vi "Auto Scorer.vi"() -> ()   [LabVIEW 2024, in "Word Search Scorer.lvlib"]
uses:
  Word Search Scorer.lvlib
  Scorer State.ctl
  Scoring Result.ctl
panel:
  out "Response":string
  out "Scoring Result":T1
  out "Run Time":dbl format="%<%M:%S%1u>t"
  out "Run Start":timestamp
  out "VI Refnum":refnum<vi>
  out "App Ref":refnum<vi>
  out "Zip":path
  out "Upload Error":errorcluster
  out "Score Error":errorcluster
  out "Download Error":errorcluster
  out "Poll Error":errorcluster
  out "Last Poll":timestamp format="%<%Y-%m-%d %H:%M:%S>T"
  out "State":T2
  out "Previous Submission":i32
  out "Current Submission":i32
  out "Time to next poll":dbl format="%#.0f"
  in  "Poll Period":dbl=60.0
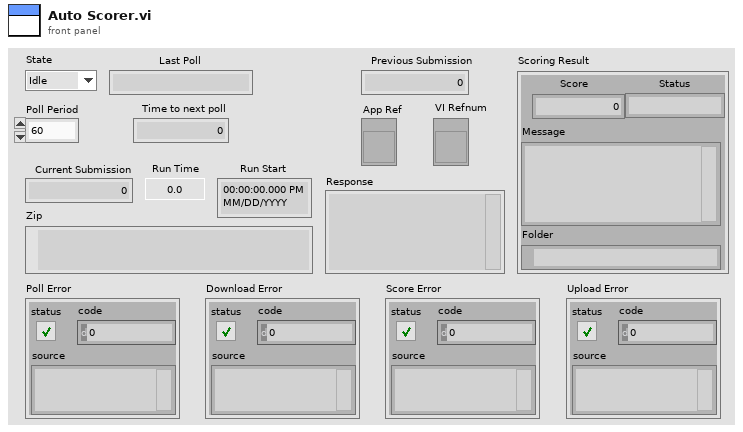
[diagram p1: front panel]
types:
  T1 = typedef "Word Search Scorer.lvlib/Scoring Result.ctl" = cluster{"Score":dbl, "Status":string, "Message":string, "Folder":path}
  T2 = typedef "Word Search Scorer.lvlib/Scorer State.ctl" = enum16{"Idle", "Poll", "Run", "Upload", "Error", "Timeout"}
  T3 = enum32{"Bad", "Idle", "Run top level", "Running"}
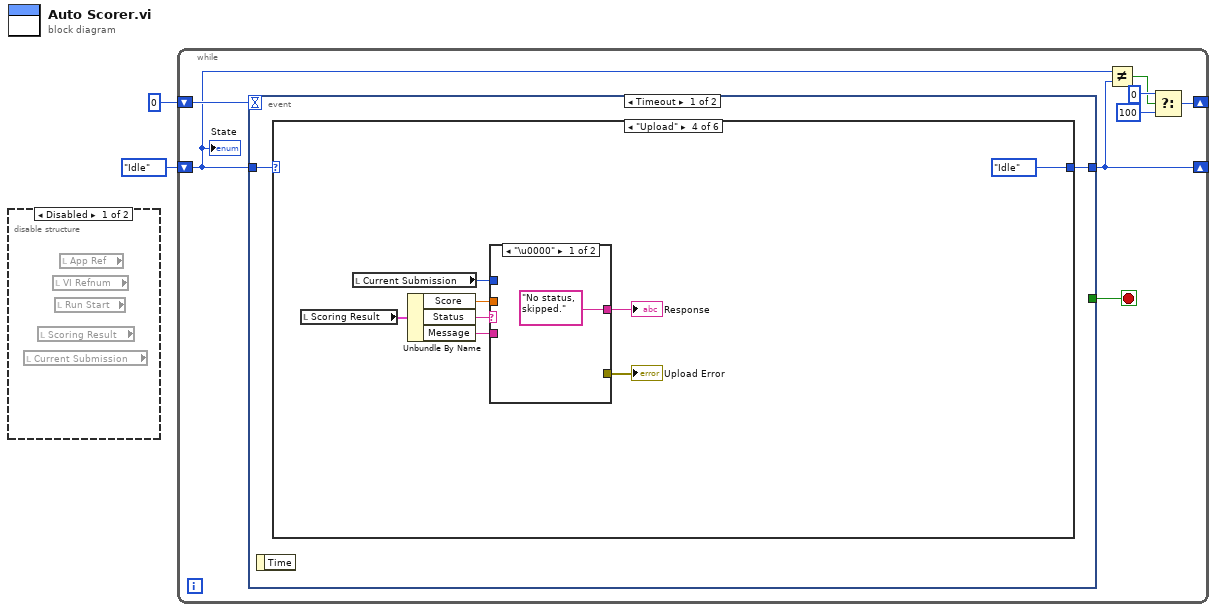
[diagram p0: block diagram]
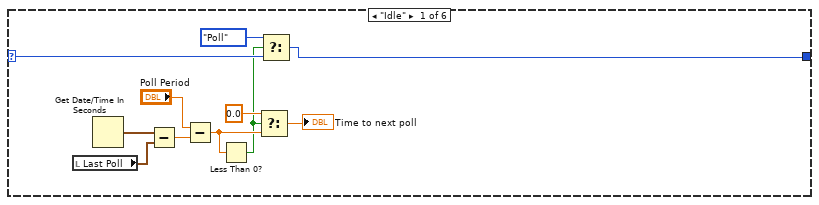
[diagram p3: hidden frame]
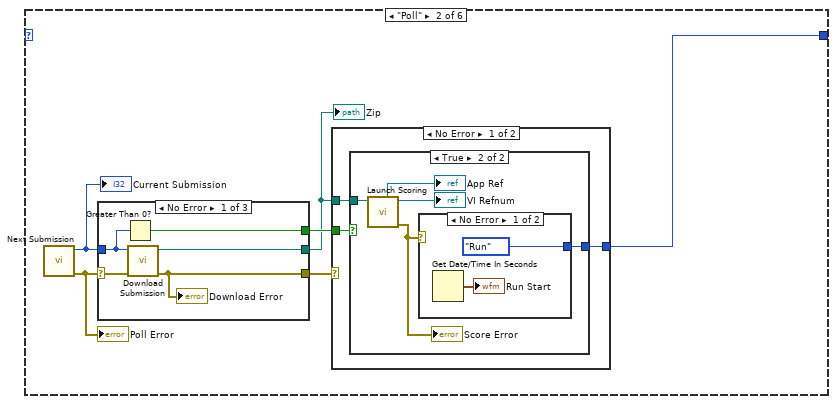
[diagram p4: hidden frame]
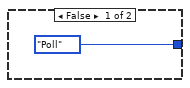
[diagram p5: hidden frame]
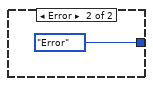
[diagram p6: hidden frame]
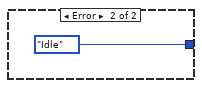
[diagram p7: hidden frame]
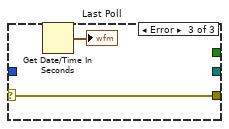
[diagram p9: hidden frame]
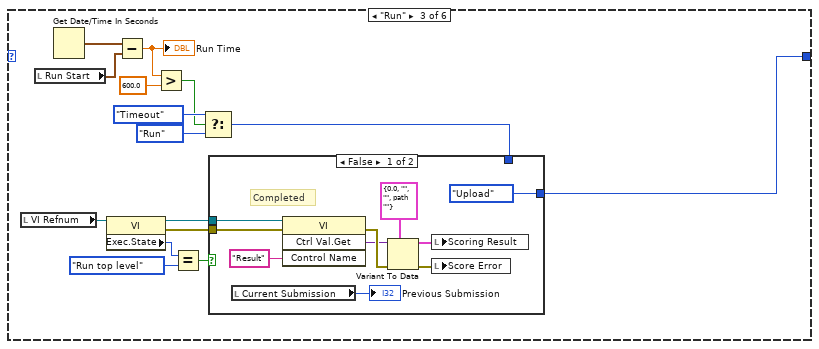
[diagram p10: hidden frame]
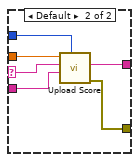
[diagram p12: hidden frame]
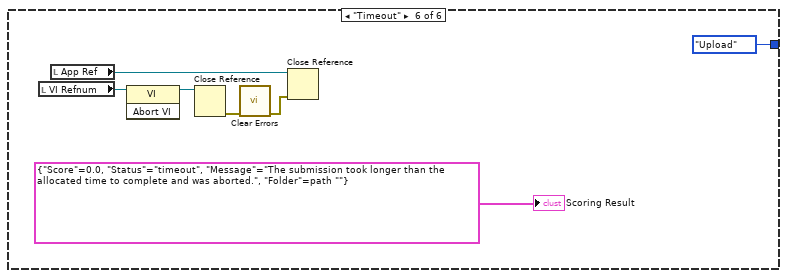
[diagram p14: hidden frame]
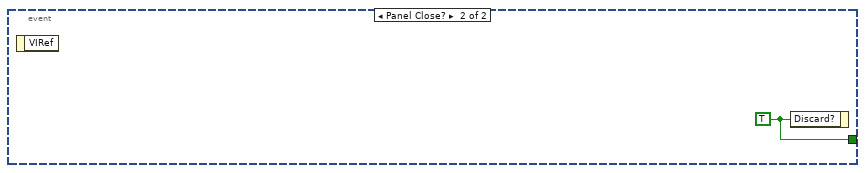
[diagram p15: hidden frame]
diagram:
  n1 = disable-structure shown="Disabled" {
    frame Disabled {
      n2 = local read "Current Submission"() -> ()  [unwired: 1 out]
      n3 = local read "Scoring Result"() -> ()  [unwired: 1 out]
      n4 = local read "VI Refnum"() -> ()  [unwired: 1 out]
      n5 = local read "Run Start"() -> ()  [unwired: 1 out]
      n6 = local read "App Ref"() -> ()  [unwired: 1 out]
    }
    frame Enabled {
    }
  }
  n7 = while {
    shift-right: [w9] -> _
    shift-left: Scorer_State."Idle" ("Scorer State") -> [w8]
    shift-right: [w6] -> _
    shift-left: 0 -> [w10]
    stop <- w3 stop-if-true
    n8 = event shown="[0] Timeout" {
      selector: _ -> [_ _]
      dyn-events: _ -> [_ _]
      timeout: w10 -> [_ _]
      tunnel: w8 -> [w12 _]
      tunnel: [w11 _] -> w9
      tunnel: [_ w100] -> w3
      event Timeout {
        n9 = event-data() -> ()  [unwired: 1 in, 1 out]
        n10 = case shown="\"Upload\"" w12 {
          selector: w12 -> [w16 _ _ _ w92 _]
          tunnel: [w13 w26 w59 Scorer_State."Idle" ("Scorer State") w92 Scorer_State."Upload" ("Scorer State")] -> w11
          frame "Idle" {
            n11 = local read "Last Poll"() -> (w22:timestamp)
            n12 = Get Date/Time In Seconds() -> (seconds since 1Jan1904=w23:timestamp)
            n13 = Subtract(x=w23, y=w22) -> (x-y=w21:dbl)
            n14 = Subtract(x="Poll Period", y=w21) -> (x-y=w19:dbl)
            n15 = Less Than 0?(x=w19) -> (x < 0?=w15:bool)
            n16 = Select(t=0.0, s=w15, f=w19) -> (s? t:f=→"Time to next poll":dbl)
            n17 = Select(t=Scorer_State."Poll", s=w15, f=w16) -> (s? t:f=w13:T2)
          }
          frame "Poll" {
            n18 = call "Next Submission.vi"() -> ("error out"=w28:errorcluster, "submission"=w24:i32)  [unwired: 9 in, 1 out]
            "Poll Error" <- w28
            "Current Submission" <- w24
            n19 = case shown="No Error" w28 {
              selector: w28 -> [w46 w48 w49]
              tunnel: w24 -> [w47 _ _]
              tunnel: [w45 _ _] -> w25
              tunnel: [w44 w48 w49] -> w29
              tunnel: [w43 _ _] -> w27
              frame No Error {
                n20 = Greater Than 0?(x=w47) -> (x > 0?=w43:bool)
                n21 = call "Download Submission.vi"("error in (no error)"=w46, "submission"=w47) -> ("error out"=w44:errorcluster, "Zip Path"=w45:path)  [unwired: 7 in, 1 out]
                "Download Error" <- w44
              }
              frame Default {
              }
              frame Error {
                # "No submissions"
                n22 = Get Date/Time In Seconds() -> (seconds since 1Jan1904=→"Last Poll":timestamp)
              }
            }
            "Zip" <- w25
            n23 = case shown="No Error" w29 {
              tunnel: w27 -> [w32 _]
              tunnel: [w31 Scorer_State."Idle" ("Scorer State")] -> w26
              tunnel: w25 -> [w30 _]
              frame No Error {
                n24 = case shown="True" w32 {
                  tunnel: [Scorer_State."Poll" ("Scorer State") w37] -> w31
                  tunnel: w30 -> [_ w34]
                  frame False {
                  }
                  frame True {
                    n25 = call "Launch Scoring.vi"("Zip"=w34) -> ("error out"=w38:errorcluster, "VI Refnum"=→"VI Refnum":refnum<vi>, "App Ref"=→"App Ref":refnum<vi>)  [unwired: 8 in]
                    "Score Error" <- w38
                    n26 = case shown="No Error" w38 {
                      tunnel: [Scorer_State."Run" ("Scorer State") Scorer_State."Error" ("Scorer State")] -> w37
                      frame No Error {
                        n27 = Get Date/Time In Seconds() -> (seconds since 1Jan1904=→"Run Start":timestamp)
                      }
                      frame Error {
                      }
                    }
                  }
                }
              }
              frame Error {
              }
            }
          }
          frame "Run" {
            n28 = local read "VI Refnum"() -> (w65:refnum<vi>)
            n29 = local read "Run Start"() -> (w61:timestamp)
            n30 = Get Date/Time In Seconds() -> (seconds since 1Jan1904=w62:timestamp)
            n31 = property class="VI"(reference=w65) -> (reference out=w52:refnum<vi>, error out=w51:errorcluster, "Exec.State"=w64:T3)  [unwired: 1 in]
            n32 = Subtract(x=w62, y=w61) -> (x-y=w58:dbl)
            "Run Time" <- w58
            n33 = Greater?(x=w58, y=600.0) -> (0:w54:bool)
            n34 = Equal?(x=w64, y=T3."Run top level") -> (x = y?=w60:bool)
            n35 = Select(t=Scorer_State."Timeout" ("Scorer State"), s=w54, f=Scorer_State."Run" ("Scorer State")) -> (s? t:f=w53:T2)
            n36 = case shown="False" w60 {
              tunnel: [Scorer_State."Upload" ("Scorer State") w76] -> w59
              tunnel: w53 -> [_ w76]
              tunnel: w52 -> [w74 _]
              tunnel: w51 -> [w71 _]
              frame False {
                # "Completed"
                n37 = local read "Current Submission"() -> (→"Previous Submission":i32)
                n38 = invoke class="VI" method="Ctrl Val.Get"(reference=w74, error in=w71, "Control Name"="Result") -> (error out=w75:errorcluster, "Get Control Value Variant"=w72:variant)  [unwired: 1 in, 2 out]
                n39 = Variant To Data(error in=w75, type=T1 {"Score"=0.0, "Status"="", "Message"="", "Folder"=path ""} ("Scoring Result"), Variant=w72) -> (data=w69:T1, error out=w68:errorcluster)
                n40 = local write "Scoring Result"(w69) -> ()
                n41 = local write "Score Error"(w68) -> ()
              }
              frame True {
                # "Still running"
              }
            }
          }
          frame "Upload" {
            n42 = local read "Scoring Result"() -> (w83:T1)
            n43 = local read "Current Submission"() -> (w81:i32)
            n44 = Unbundle By Name(w83) -> ("Score"=w82:dbl, "Status"=w80:string, "Message"=w79:string)
            n45 = case shown="\"\"" w80 {
              selector: w80 -> [_ w89]
              tunnel: w82 -> [_ w91]
              tunnel: w81 -> [_ w90]
              tunnel: w79 -> [_ w88]
              tunnel: [_ w87] -> w78
              tunnel: ["No status, skipped." ("Response") w86] -> w77
              frame "\u0000" {
              }
              frame Default {
                n46 = call "Upload Score.vi"("submission"=w90, "result"=w88, "status"=w89, "Run Time"=w91) -> ("error out"=w87:errorcluster, "Response"=w86:string)  [unwired: 5 in, 1 out]
              }
            }
            "Upload Error" <- w78
            "Response" <- w77
          }
          frame "Error" {
            # "Whoops! Time to be saved!"
          }
          frame "Timeout" {
            n47 = local read "VI Refnum"() -> (w97:refnum<vi>)
            n48 = local read "App Ref"() -> (w93:refnum<vi>)
            n49 = invoke class="VI" method="Abort VI"(reference=w97) -> (reference out=w96:refnum<vi>)  [unwired: 2 in, 2 out]
            n50 = Close Reference(reference=w96) -> (error out=w95:errorcluster)  [unwired: 1 in]
            n51 = call <vilib>:"Clear Errors.vi"("error in (no error)"=w95) -> ("error out"=w94:errorcluster)  [unwired: 5 in, 1 out]
            n52 = Close Reference(reference=w93, error in (no error)=w94) -> ()  [unwired: 1 out]
            "Scoring Result" <- T1 {"Score"=0.0, "Status"="timeout", "Message"="The submission took longer than the allocated time to complete and was aborted.", "Folder"=path ""} ("Scoring Result")
          }
        }
      }
      event Panel Close? {
        w100 = TRUE ("Discard?")
        n53 = event-data() -> ()  [unwired: 1 in, 1 out]
        n54 = event-data("Discard?"=w100) -> ()  [unwired: 1 in, 1 out]
      }
    }
    n55 = Not Equal?(x=w8, y=w9) -> (x != y?=w4:bool)
    n56 = Select(t=0, s=w4, f=100) -> (s? t:f=w6:i32)
    "State" <- w8
  }
